vi "LINEAR REGRESSION.vi"() -> ()   [LabVIEW 2018]
uses:
  <vilib>/Analysis/1siggen.llb/Ramp Pattern by Samples.vi
  <vilib>/Analysis/NI_AALBase.lvlib
  <vilib>/Analysis/NI_AALPro.lvlib
panel:
  out "Ramp Pattern 8":dbl[](array[numeric])
  out "slope 7":dbl
  out "intercept 7":dbl
  in  "element":dbl
  out "Ramp Pattern 7":dbl[](array[numeric])
  out "Waveform Graph 2":dbl[](graph)
  out "Waveform Graph":dbl[](graph)
  out "x+y 2":dbl
  out "x+y":dbl
  out "Ramp Pattern 6":dbl[](array[numeric])
  out "XY Graph 6":T1(graph)
  out "slope 6":dbl
  out "intercept 6":dbl
  out "Ramp Pattern 5":dbl[](array[numeric])
  out "slope 5":dbl
  out "intercept 5":dbl
  out "appended array":dbl[][](array[numeric])
  out "Ramp Pattern 4":dbl[](array[numeric])
  out "slope 4":dbl
  out "intercept 4":dbl
  out "Ramp Pattern 3":dbl[](array[numeric])
  out "slope 3":dbl
  out "intercept 3":dbl
  out "Ramp Pattern 2":dbl[](array[numeric])
  out "slope 2":dbl
  out "intercept 2":dbl
  out "intercept":dbl
  out "slope":dbl
  out "Ramp Pattern":dbl[](array[numeric])
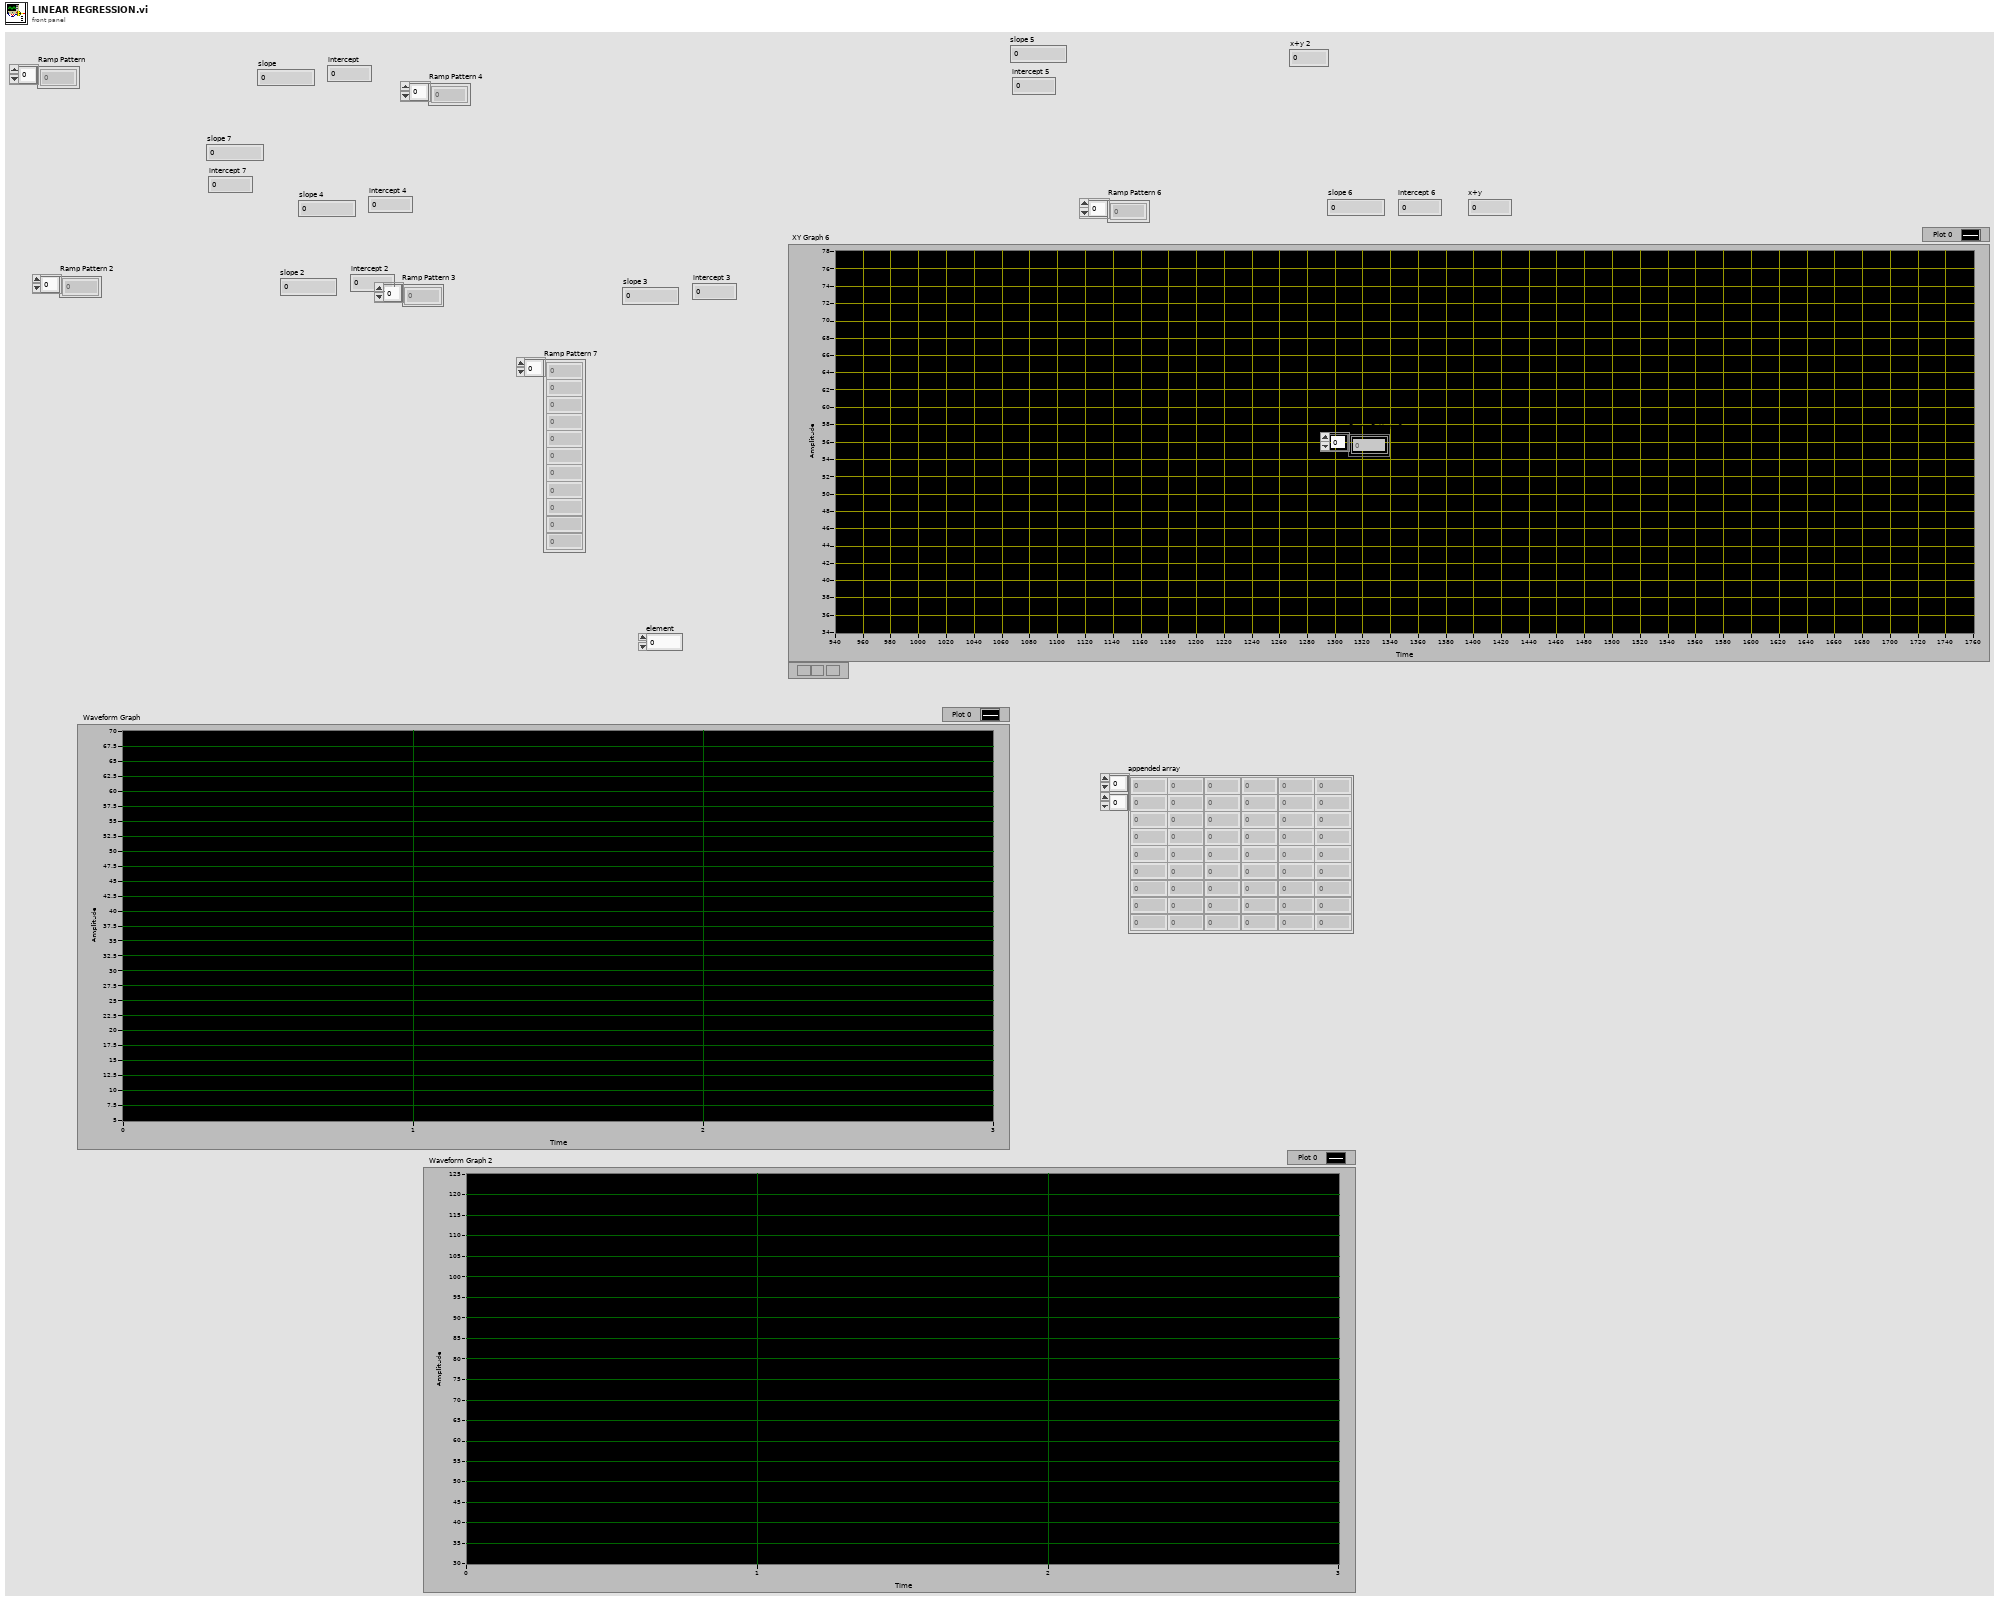
[diagram p1: front panel]
types:
  T1 = cluster{"Ramp Pattern":dbl[], "Ramp Pattern":dbl[]}
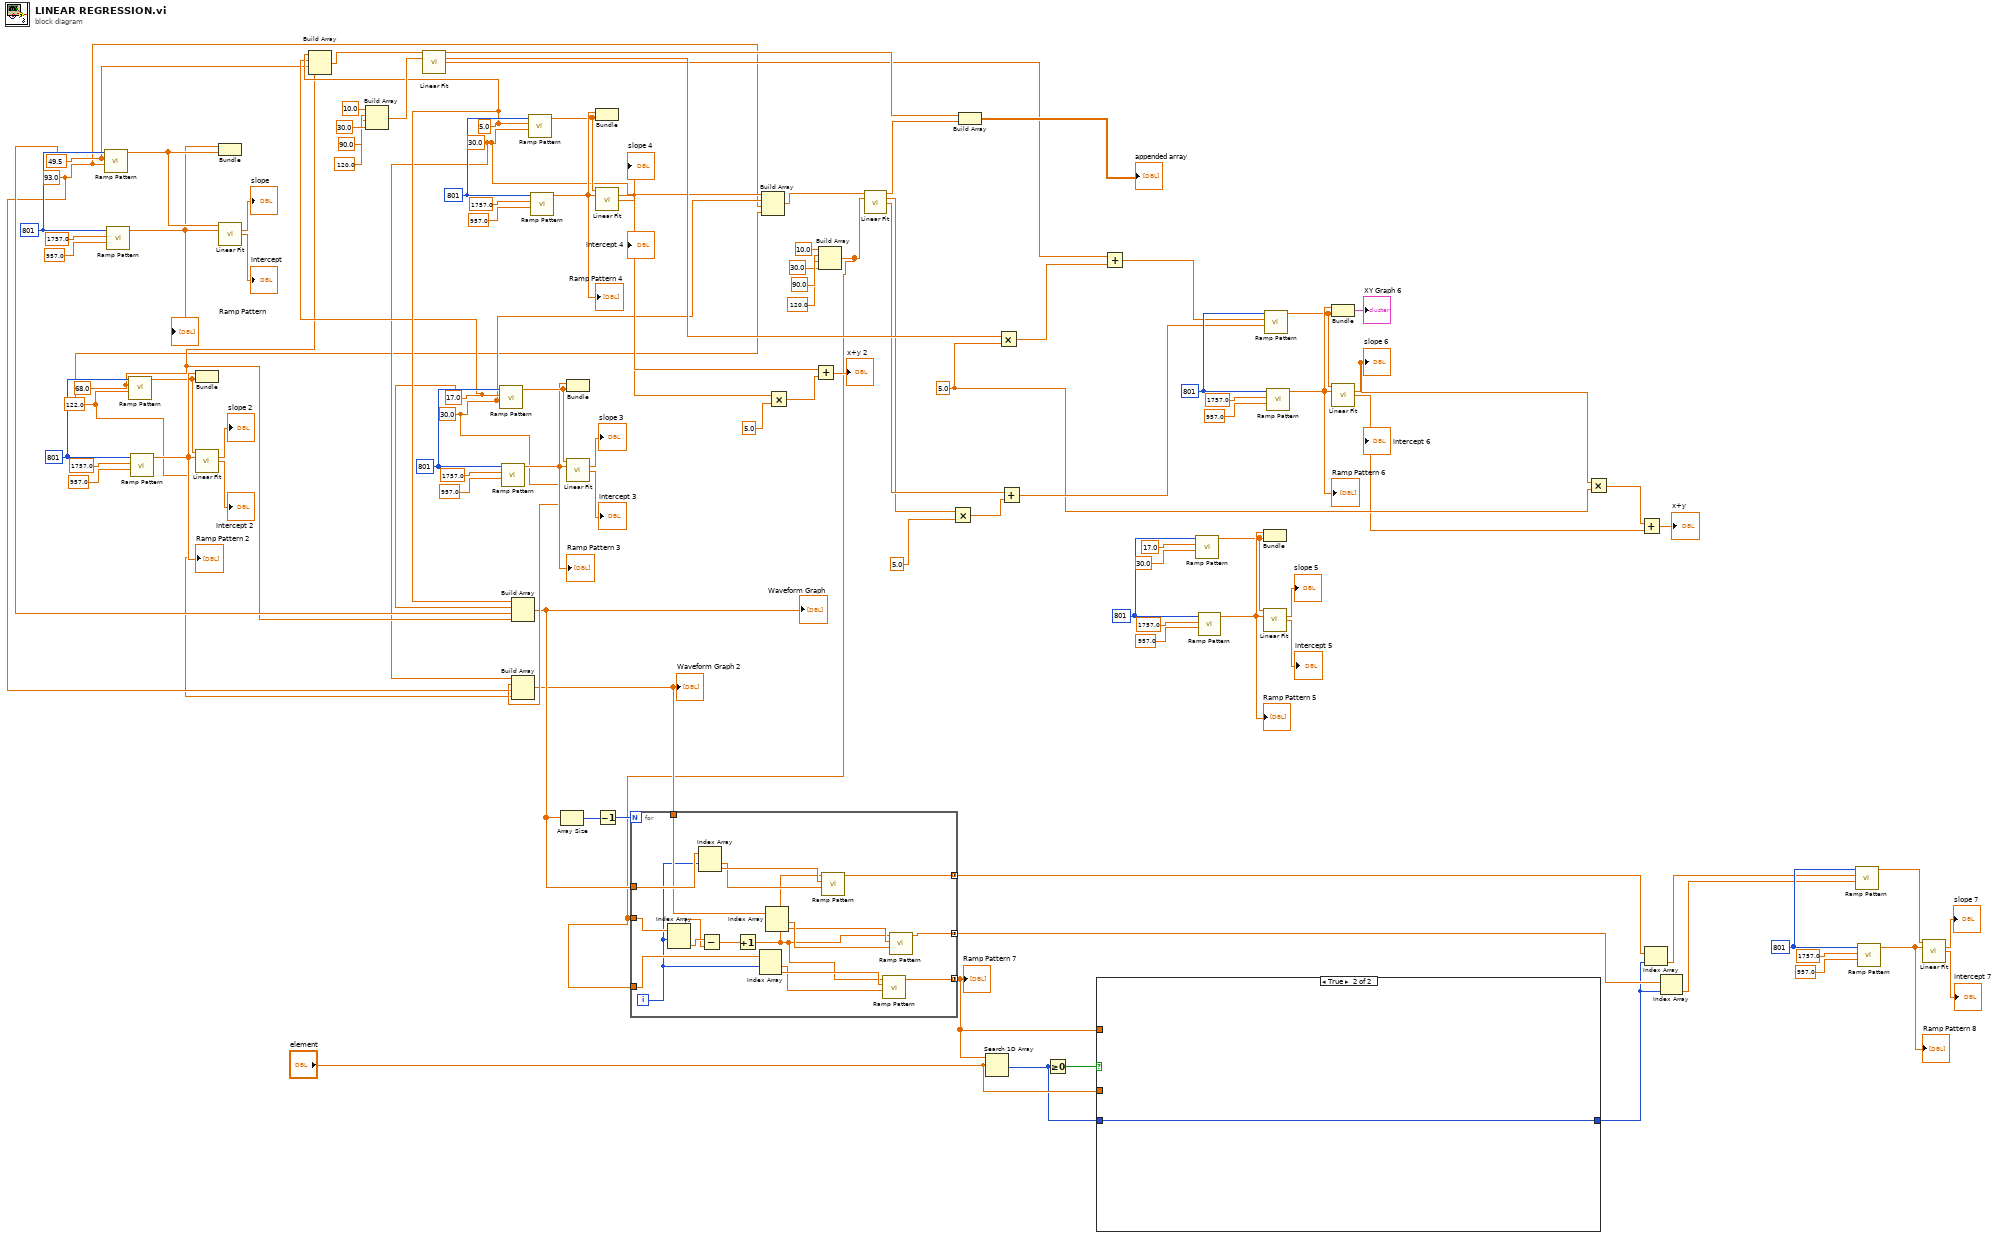
[diagram p0: block diagram]
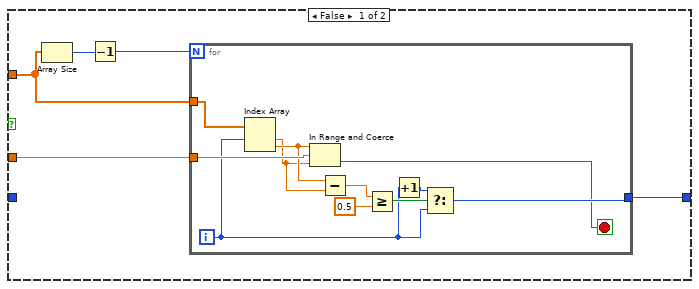
[diagram p2: hidden frame]
diagram:
  w8 = 801 ("samples")
  w44 = 801 ("samples")
  w54 = 801 ("samples")
  w38 = 5.0 ("element")
  w29 = 5.0 ("end")
  w25 = 30.0 ("start")
  w80 = 801 ("samples")
  w28 = 17.0 ("end")
  w24 = 30.0 ("start")
  w87 = 801 ("samples")
  w26 = 68.0 ("end")
  w22 = 122.0 ("start")
  w92 = 801 ("samples")
  w27 = 49.5 ("end")
  w23 = 93.0 ("start")
  w101 = 801 ("samples")
  n1 = call-poly <vilib>:"Ramp Pattern.vi"("start"=w23, "end"=w27, "samples"=w101) -> ("Ramp Pattern"=w100:dbl[])  [unwired: 7 in, 1 out]
  n2 = call-poly <vilib>:"Ramp Pattern.vi"("start"=957.0, "end"=1757.0, "samples"=w101) -> ("Ramp Pattern"=w99:dbl[])  [unwired: 7 in, 1 out]
  "Ramp Pattern" <- w99
  n3 = call-poly <vilib>:"Ramp Pattern.vi"("start"=w22, "end"=w26, "samples"=w92) -> ("Ramp Pattern"=w93:dbl[])  [unwired: 7 in, 1 out]
  n4 = call-poly <vilib>:"Ramp Pattern.vi"("start"=957.0, "end"=1757.0, "samples"=w92) -> ("Ramp Pattern"=w94:dbl[])  [unwired: 7 in, 1 out]
  "Ramp Pattern 2" <- w94
  n5 = Bundle("Ramp Pattern"=w94, "Ramp Pattern"=w93) -> ()  [unwired: 1 in, 1 out]
  n6 = call <vilib>:"Linear Fit.vi"("Y"=w93, "X"=w94) -> ("slope"=→"slope 2":dbl, "intercept"=→"intercept 2":dbl)  [unwired: 9 in, 3 out]
  n7 = Bundle("Ramp Pattern"=w99, "Ramp Pattern"=w100) -> ()  [unwired: 1 in, 1 out]
  n8 = call <vilib>:"Linear Fit.vi"("Y"=w100, "X"=w99) -> ("slope"=→"slope":dbl, "intercept"=→"intercept":dbl)  [unwired: 9 in, 3 out]
  n9 = Build Array(w29, w28, w27, w26) -> (w73:dbl[])
  n10 = Build Array(10.0 ("element"), 120.0 ("element"), 90.0 ("element"), 30.0 ("element")) -> (w72:dbl[])
  n11 = call <vilib>:"Linear Fit.vi"("Y"=w73, "X"=w72) -> ("Best Linear Fit"=w66:dbl[], "slope"=w63:dbl, "intercept"=w61:dbl)  [unwired: 9 in, 2 out]
  n12 = call-poly <vilib>:"Ramp Pattern.vi"("start"=w24, "end"=w28, "samples"=w87) -> ("Ramp Pattern"=w86:dbl[])  [unwired: 7 in, 1 out]
  n13 = call-poly <vilib>:"Ramp Pattern.vi"("start"=957.0, "end"=1757.0, "samples"=w87) -> ("Ramp Pattern"=w85:dbl[])  [unwired: 7 in, 1 out]
  "Ramp Pattern 3" <- w85
  n14 = Build Array(w29, w28, w27, w26) -> (w19:dbl[])
  "Waveform Graph" <- w19
  n15 = Build Array(w25, w24, w23, w22) -> (w18:dbl[])
  "Waveform Graph 2" <- w18
  n16 = call-poly <vilib>:"Ramp Pattern.vi"("start"=w25, "end"=w29, "samples"=w80) -> ("Ramp Pattern"=w81:dbl[])  [unwired: 7 in, 1 out]
  n17 = call-poly <vilib>:"Ramp Pattern.vi"("start"=957.0, "end"=1757.0, "samples"=w80) -> ("Ramp Pattern"=w82:dbl[])  [unwired: 7 in, 1 out]
  "Ramp Pattern 4" <- w82
  n18 = Array Size(array=w19) -> (size(s)=w21:i32)
  n19 = Bundle("Ramp Pattern"=w85, "Ramp Pattern"=w86) -> ()  [unwired: 1 in, 1 out]
  n20 = call <vilib>:"Linear Fit.vi"("Y"=w86, "X"=w85) -> ("slope"=→"slope 3":dbl, "intercept"=→"intercept 3":dbl)  [unwired: 9 in, 3 out]
  n21 = Bundle("Ramp Pattern"=w82, "Ramp Pattern"=w81) -> ()  [unwired: 1 in, 1 out]
  n22 = call <vilib>:"Linear Fit.vi"("Y"=w81, "X"=w82) -> ("slope"=w32:dbl, "intercept"=w33:dbl)  [unwired: 9 in, 3 out]
  "slope 4" <- w32
  "intercept 4" <- w33
  n23 = Decrement(x=w21) -> (x-1=w20:i32)
  n24 = Build Array(w25, w24, w23, w22) -> (w71:dbl[])
  n25 = Multiply(x=w32, y=5.0) -> (x*y=w34:dbl)
  n26 = Add(x=w33, y=w34) -> (x+y=→"x+y 2":dbl)
  n27 = Build Array(10.0 ("element"), 120.0 ("element"), 90.0 ("element"), 30.0 ("element")) -> (w17:dbl[])
  n28 = for {
    N: w20 -> [_]
    tunnel: w19 -> [w117]
    tunnel: w18 -> [w112]
    tunnel: w17 -> [w121]
    tunnel: [w118] -> w12 mode=concatenating
    tunnel: [w111] -> w11 mode=concatenating
    tunnel: w17 -> [w108]
    tunnel: [w105] -> w15 mode=concatenating
    i -> [w107]
    n29 = Index Array(array=w121, index #1=w107) -> (element #1=w119:dbl, element #2=w120:dbl)  [unwired: 1 in]
    n30 = Index Array(array=w117, index #1=w107) -> (element #1=w115:dbl, element #2=w116:dbl)  [unwired: 1 in]
    n31 = Subtract(x=w120, y=w119) -> (x-y=w106:dbl)
    n32 = Increment(x=w106) -> (x+1=w104:dbl)
    n33 = Index Array(array=w108, index #1=w107) -> (element #1=w109:dbl, element #2=w110:dbl)  [unwired: 1 in]
    n34 = Index Array(array=w112) -> (element #1=w114:dbl, element #2=w113:dbl)  [unwired: 2 in]
    n35 = call-poly <vilib>:"Ramp Pattern.vi"("start"=w115, "end"=w116, "samples"=w104) -> ("Ramp Pattern"=w118:dbl[])  [unwired: 7 in, 1 out]
    n36 = call-poly <vilib>:"Ramp Pattern.vi"("start"=w109, "end"=w110, "samples"=w104) -> ("Ramp Pattern"=w105:dbl[])  [unwired: 7 in, 1 out]
    n37 = call-poly <vilib>:"Ramp Pattern.vi"("start"=w114, "end"=w113, "samples"=w104) -> ("Ramp Pattern"=w111:dbl[])  [unwired: 7 in, 1 out]
  }
  "Ramp Pattern 7" <- w15
  n38 = call <vilib>:"Linear Fit.vi"("Y"=w71, "X"=w17) -> ("Best Linear Fit"=w65:dbl[], "slope"=w48:dbl, "intercept"=w49:dbl)  [unwired: 9 in, 2 out]
  n39 = Multiply(x=w48, y=5.0 ("element")) -> (x*y=w51:dbl)
  n40 = Build Array(w66, w65) -> (→"appended array":dbl[][])
  n41 = Search 1D Array(1D array=w15, element="element") -> (index of element=w13:i32)  [unwired: 1 in]
  n42 = Multiply(x=w63, y=w38) -> (x*y=w62:dbl)
  n43 = Add(x=w49, y=w51) -> (x+y=w40:dbl)
  n44 = Greater Or Equal To 0?(x=w13) -> (x >= 0?=w16:bool)
  n45 = case shown="True" w16 {
    tunnel: w15 -> [w124 _]
    tunnel: "element" -> [w123 _]
    tunnel: [w122 w138] -> w3
    tunnel: w13 -> [_ w138]
    frame False {
      n46 = Array Size(array=w124) -> (size(s)=w126:i32)
      n47 = Decrement(x=w126) -> (x-1=w125:i32)
      n48 = for {
        N: w125 -> [_]
        tunnel: w124 -> [w137]
        tunnel: w123 -> [w136]
        tunnel: [w128] -> w122
        i -> [w130]
        stop <- w127 stop-if-true
        n49 = Index Array(array=w137, index #1=w130) -> (element #1=w131:dbl, element #2=w132:dbl)  [unwired: 1 in]
        n50 = In Range and Coerce(upper limit=w132, x=w136, lower limit=w131) -> (In Range?=w127:bool)  [unwired: 1 out]
        n51 = Subtract(x=w132, y=w131) -> (x-y=w135:dbl)
        n52 = Greater Or Equal?(x=w135, y=0.5) -> (x >= y?=w133:bool)
        n53 = Increment(x=w130) -> (x+1=w129:i32)
        n54 = Select(t=w129, s=w133, f=w130) -> (s? t:f=w128:i32)
      }
    }
    frame True {
    }
  }
  n55 = Add(x=w61, y=w62) -> (x+y=w41:dbl)
  n56 = call-poly <vilib>:"Ramp Pattern.vi"("start"=30.0, "end"=17.0, "samples"=w54) -> ("Ramp Pattern"=w55:dbl[])  [unwired: 7 in, 1 out]
  n57 = call-poly <vilib>:"Ramp Pattern.vi"("start"=957.0, "end"=1757.0, "samples"=w54) -> ("Ramp Pattern"=w56:dbl[])  [unwired: 7 in, 1 out]
  "Ramp Pattern 5" <- w56
  n58 = Bundle("Ramp Pattern"=w56, "Ramp Pattern"=w55) -> ()  [unwired: 1 in, 1 out]
  n59 = call <vilib>:"Linear Fit.vi"("Y"=w55, "X"=w56) -> ("slope"=→"slope 5":dbl, "intercept"=→"intercept 5":dbl)  [unwired: 9 in, 3 out]
  n60 = call-poly <vilib>:"Ramp Pattern.vi"("start"=w40, "end"=w41, "samples"=w44) -> ("Ramp Pattern"=w46:dbl[])  [unwired: 7 in, 1 out]
  n61 = call-poly <vilib>:"Ramp Pattern.vi"("start"=957.0, "end"=1757.0, "samples"=w44) -> ("Ramp Pattern"=w47:dbl[])  [unwired: 7 in, 1 out]
  "Ramp Pattern 6" <- w47
  n62 = Bundle("Ramp Pattern"=w47, "Ramp Pattern"=w46) -> (→"XY Graph 6":T1)  [unwired: 1 in]
  n63 = call <vilib>:"Linear Fit.vi"("Y"=w46, "X"=w47) -> ("slope"=w39:dbl, "intercept"=w36:dbl)  [unwired: 9 in, 3 out]
  "slope 6" <- w39
  "intercept 6" <- w36
  n64 = Multiply(x=w39, y=w38) -> (x*y=w37:dbl)
  n65 = Add(x=w37, y=w36) -> (x+y=→"x+y":dbl)
  n66 = Index Array(array=w12, index=w3) -> (element=w2:dbl)
  n67 = Index Array(array=w11, index=w3) -> (element=w1:dbl)
  n68 = call-poly <vilib>:"Ramp Pattern.vi"("start"=w1, "end"=w2, "samples"=w8) -> ("Ramp Pattern"=w7:dbl[])  [unwired: 7 in, 1 out]
  n69 = call-poly <vilib>:"Ramp Pattern.vi"("start"=957.0, "end"=1757.0, "samples"=w8) -> ("Ramp Pattern"=w6:dbl[])  [unwired: 7 in, 1 out]
  "Ramp Pattern 8" <- w6
  n70 = call <vilib>:"Linear Fit.vi"("Y"=w7, "X"=w6) -> ("slope"=→"slope 7":dbl, "intercept"=→"intercept 7":dbl)  [unwired: 9 in, 3 out]
